vi "Read Save_.vi"(8 "error in (no error)":errorcluster, 11 "Change File Writing State MSG in":refnum<class "Change File Writing State MSG.lvclass">) -> (0 "error out":errorcluster, 2 "Save?":bool, 3 "Change File Writing State MSG out":refnum<class "Change File Writing State MSG.lvclass">)   [LabVIEW 2017, in "File Library.lvlib" / "Change File Writing State MSG.lvclass"]
uses:
  Change File Writing State MSG.lvclass
  Change File Writing State MSG.lvclass/Change File Writing State MSG.ctl
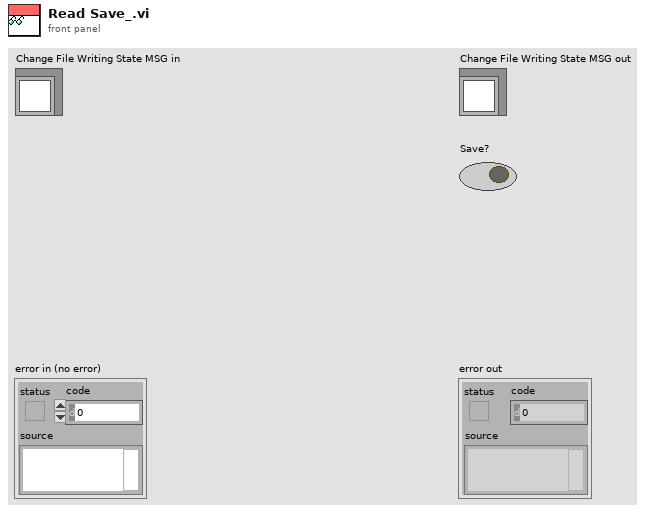
[diagram p1: front panel]
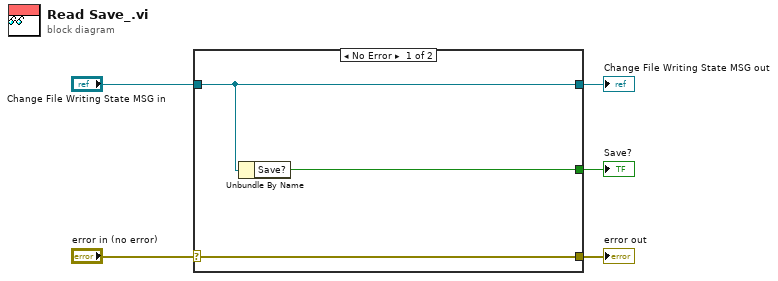
[diagram p0: block diagram]
diagram:
  n1 = case shown="No Error" "error in (no error)" {
    selector: "error in (no error)" -> [w8 w9]
    tunnel: [w8 w9] -> w4
    tunnel: [w7 w10] -> w2
    tunnel: "Change File Writing State MSG in" -> [w7 w10]
    tunnel: [w6 _] -> w1
    frame No Error {
      n2 = Unbundle By Name(w7) -> ("Save?"=w6:bool)
    }
    frame Error {
    }
  }
  "error out" <- w4
  "Change File Writing State MSG out" <- w2
  "Save?" <- w1
